vi "OFF64.vi"(1 "lines":tag="Dev2/port0/line0:7") -> (0 "Status(U8)":u8)   [LabVIEW 2020]
uses:
  <vilib>/DAQmx/write.llb/DAQmx Write (Digital U8 1Chan 1Samp).vi
  <vilib>/DAQmx/create/channels.llb/DAQmx Create Channel (DO-Digital Output).vi
  <vilib>/DAQmx/miscellaneous.llb/DAQmx Fill In Error Info.vi
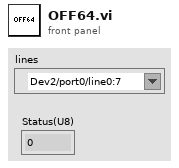
[diagram p1: front panel]
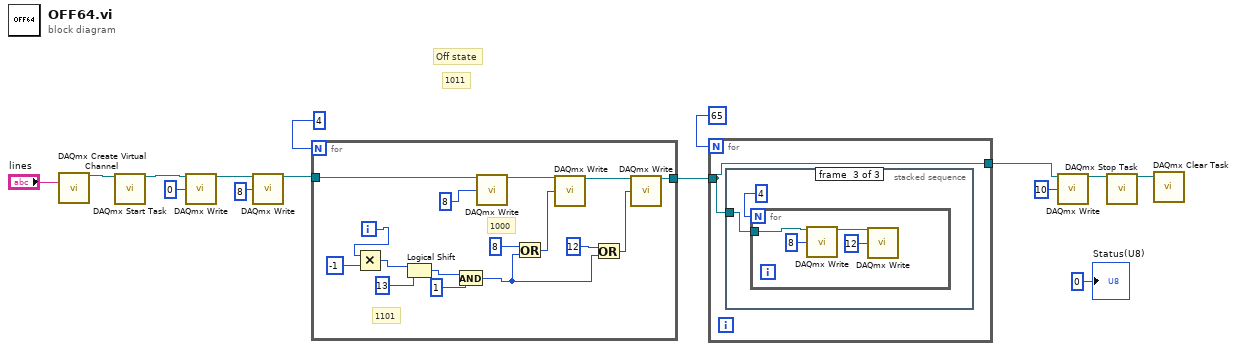
[diagram p0: block diagram]
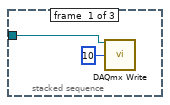
[diagram p2: hidden frame]
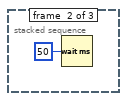
[diagram p3: hidden frame]
diagram:
  # "Off state"
  # "1011"
  n1 = call-poly <vilib>:"DAQmx Create Virtual Channel.vi"("lines"="lines") -> ("task out"=w15:refnum<k21>)  [unwired: 13 in, 1 out]
  n2 = call <vilib>:"DAQmx Start Task.vi"("task/channels in"=w15) -> ("task out"=w7:refnum<k21>)  [unwired: 13 in, 1 out]
  n3 = call-poly <vilib>:"DAQmx Write.vi"("task/channels in"=w7, "data"=u8 0) -> ("task out"=w6:refnum<k21>)  [unwired: 11 in, 2 out]
  n4 = call-poly <vilib>:"DAQmx Write.vi"("task/channels in"=w6, "data"=u8 8) -> ("task out"=w11:refnum<k21>)  [unwired: 11 in, 2 out]
  n5 = for {
    N: 4 -> [_]
    tunnel: w11 -> [w20]
    tunnel: [w17] -> w3
    i -> [w29]
    # "1000"
    # "1101"
    n6 = Multiply(x=w29, y=-1) -> (x*y=w27:i32)
    n7 = Logical Shift(y=w27, x=u8 13) -> (x << y=w31:u8)
    n8 = And(x=w31, y=u32 1) -> (x .and. y?=w23:u32)
    n9 = call-poly <vilib>:"DAQmx Write.vi"("task/channels in"=w20, "data"=u32 8 ("x")) -> ("task out"=w19:refnum<k21>)  [unwired: 11 in, 2 out]
    n10 = Or(x=u32 8, y=w23) -> (x .or. y?=w24:u32)
    n11 = call-poly <vilib>:"DAQmx Write.vi"("task/channels in"=w19, "data"=w24) -> ("task out"=w18:refnum<k21>)  [unwired: 11 in, 2 out]
    n12 = Or(x=u32 12, y=w23) -> (x .or. y?=w21:u32)
    n13 = call-poly <vilib>:"DAQmx Write.vi"("task/channels in"=w18, "data"=w21) -> ("task out"=w17:refnum<k21>)  [unwired: 11 in, 2 out]
  }
  n14 = for {
    N: 65 -> [_]
    tunnel: w3 -> [w32]
    tunnel: [w32] -> w2
    n15 = stacked-sequence {
      tunnel: w32 -> [w33 _ w36]
      frame #0 {
        n16 = call-poly <vilib>:"DAQmx Write.vi"("task/channels in"=w33, "data"=u8 10) -> ()  [unwired: 11 in, 3 out]
      }
      frame #1 {
        n17 = Wait (ms)(milliseconds to wait=u32 50) -> ()  [unwired: 1 out]
      }
      frame #2 {
        n18 = for {
          N: 4 -> [_]
          tunnel: w36 -> [w39]
          n19 = call-poly <vilib>:"DAQmx Write.vi"("task/channels in"=w39, "data"=u8 8) -> ("task out"=w38:refnum<k21>)  [unwired: 11 in, 2 out]
          n20 = call-poly <vilib>:"DAQmx Write.vi"("task/channels in"=w38, "data"=u8 12) -> ()  [unwired: 11 in, 3 out]
        }
      }
    }
  }
  n21 = call-poly <vilib>:"DAQmx Write.vi"("task/channels in"=w2, "data"=u8 10) -> ("task out"=w10:refnum<k21>)  [unwired: 11 in, 2 out]
  n22 = call <vilib>:"DAQmx Stop Task.vi"("task/channels in"=w10) -> ("task out"=w14:refnum<k21>)  [unwired: 13 in, 1 out]
  n23 = call <vilib>:"DAQmx Clear Task.vi"("task in"=w14) -> ()  [unwired: 14 in, 1 out]
  "Status(U8)" <- u8 0
